vi "Set Valve State.vi"(0 "reference in":refnum<class "FPGA API.lvclass">, 5 "#DO":T1[](array[typedef]) items=["DO 0 [KP1] [M12]", "DO 1 [ON KP2] [M21]", "DO 2 [ON KP3] [M24]", "DO 3 [WATER Y18.1 [DO3]]", "DO 4 [WATER Y18.2 [DO4]]", "DO 5 [KP6 Y29.1 33.7]", "DO 6 [KP7 Y29.2 33.8]", "DO 7 [KP8 Y29.3 33.9]", "DO 8 [KP9 Y29.4  33.12]", "DO 9 [KP10 Y29.5 33.1]", "DO 10 [KP11 Y29.6 33.2]", "DO 11 [KP12 Y29.7  33.13]", "DO 12 [KP13 Y29.8  33.11]", "DO 13 [KP14 Y29.9 33.10]", "DO 14 [KP15 Y29.10  33.6]", "DO 15 [KP16 Y29.11  33.5]", "DO 16 [KP17 Y29.12  33.4]", "DO 17 [KP18 Y29.13 33.3]", "DO 18 [AIR KP19]", "DO 19 [STEP DRIVE EN KP20]", "DO 20 [KP21 Y44.1 OPEN]", "DO 21 [ KP22 Y44.1 CLOSE]", "DO 22 [ KP23 Y44.2 OPEN]", "DO 23", "DO 24 [STEP DRIVE 1]", "DO 25 [STEP DRIVE 2]"], 7 "Time uSec":u32, 11 "error in (no error)":errorcluster) -> (4 "reference out":refnum<class "FPGA API.lvclass">, 15 "error out":errorcluster)   [LabVIEW 2019, in "Stand.lvclass"]
uses:
  Stand.lvclass
  FPGA_API_class/FPGA API.lvclass
  FPGA/TypeDef/DO index.ctl
  628819af-fd07-4303-9780-3ddd467101db.vi
  e7d2c9dc-ba67-4685-b926-bcce34aa2778.vi
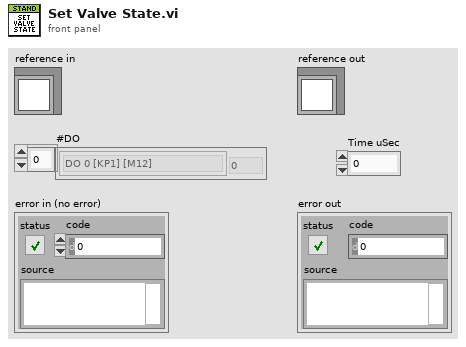
[diagram p1: front panel]
types:
  T1 = typedef "DO index.ctl" = u8
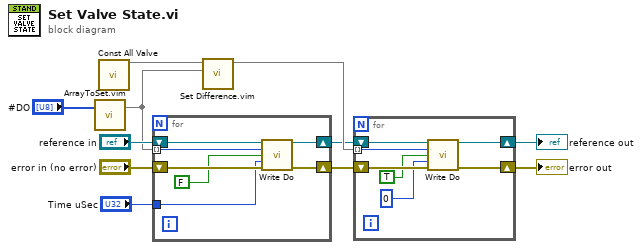
[diagram p0: block diagram]
diagram:
  n1 = call "ArrayToSet.vim"("Array"="#DO") -> ("Set"=w8:set{T1})  [unwired: 2 in]
  n2 = call "Const All Valve.vi"() -> ("Set"=w11:set{T1})  [unwired: 15 in]
  n3 = for {
    shift-right: [w16] -> w4
    shift-left: "error in (no error)" -> [w17]
    tunnel: w8 -> [w15] mode=indexing
    shift-right: [w13] -> w3
    shift-left: "reference in" -> [w18]
    tunnel: "Time uSec" -> [w12]
    n4 = call-dynamic "Write Do.vi"("FPGA API in"=w18, "#DO"=w15, "value"=FALSE, "Time uSec"=w12, "error in (no error)"=w17) -> ("FPGA API out"=w13:refnum<class "FPGA API.lvclass">, "error out"=w16:errorcluster)  [unwired: 9 in]
  }
  n5 = call "Set Difference.vim"("set 2"=w8, "set 1"=w11) -> ("difference"=w9:set{T1})  [unwired: 9 in]
  n6 = for {
    shift-right: [w23] -> w6
    shift-left: w4 -> [w24]
    tunnel: w9 -> [w22] mode=indexing
    shift-right: [w19] -> w5
    shift-left: w3 -> [w25]
    n7 = call-dynamic "Write Do.vi"("FPGA API in"=w25, "#DO"=w22, "value"=TRUE, "Time uSec"=u32 0, "error in (no error)"=w24) -> ("FPGA API out"=w19:refnum<class "FPGA API.lvclass">, "error out"=w23:errorcluster)  [unwired: 9 in]
  }
  "error out" <- w6
  "reference out" <- w5
